vi "Z900_navX_Internal_Open.vi"(8 "error in":errorcluster, 11 "navX Device":T1={"Interface"={"Protocol"=enum."SERIAL", "Update Rate (4Hz-60Hz)"=4, "navX Open TypeDef"=variant}, "Notify Packet"=refnum, "Loop VI Refnum"=refnum, "Ready to Close Occurrence Refnum"=refnum} {"Interface"."Update Rate (4Hz-60Hz)" min=4 max=60 step=1}) -> (0 "error out":errorcluster, 2 "Interface TypeDefs":T3 {"I2CDevRef"."Device Address" format="%.0x"}, 3 "navX Device":T1={"Interface"={"Protocol"=enum."SERIAL", "Update Rate (4Hz-60Hz)"=4, "navX Open TypeDef"=variant}, "Notify Packet"=refnum, "Loop VI Refnum"=refnum, "Ready to Close Occurrence Refnum"=refnum} {"Interface"."Update Rate (4Hz-60Hz)" min=4 max=60 step=1})   [LabVIEW 2016, in "navX Library v2.lvlib"]
doc: "This navX VI handles opening the Serial/I2C/SPI reference for the navX.\nTHIS VI SHOULD NOT BE CALLED BY THE USER!"
uses:
  navX Library v2.lvlib
  TypeDefs/Z900_navX_DeviceTypeDef.ctl
  TypeDefs/Z900_navX_ProtocolTypeDef.ctl
  TypeDefs/Z900_navX_NotifyPacketTypeDef.ctl
  TypeDefs/Z900_navX_ActionTypeDef.ctl
  TypeDefs/Z900_navX_InterfaceTypeDef.ctl
  <vilib>/Rock Robotics/WPI/SerialPort/WPI_SerialPortRef.ctl
  <vilib>/Rock Robotics/WPI/I2C/WPI_I2CDevRef.ctl
  <vilib>/Rock Robotics/SystemInterfaces/i2clib/i2c_bus.ctl
  <vilib>/Rock Robotics/WPI/SPI/WPI_SPIDevRef.ctl
  <vilib>/Rock Robotics/SystemInterfaces/spilib/spi_bus.ctl
  TypeDefs/navX Open TypeDefs/Z900_navX_OpenTypeDef_Serial.ctl
  NI WPI/WPI_SerialPort_USB.ctl
  TypeDefs/Z900_navX_SerialStreamTypeDef.ctl
  TypeDefs/navX Open TypeDefs/Z900_navX_OpenTypeDef_I2C.ctl
  TypeDefs/navX Open TypeDefs/Z900_navX_OpenTypeDef_SPI.ctl
  NI WPI/NI WPI Serial USB.lvlib
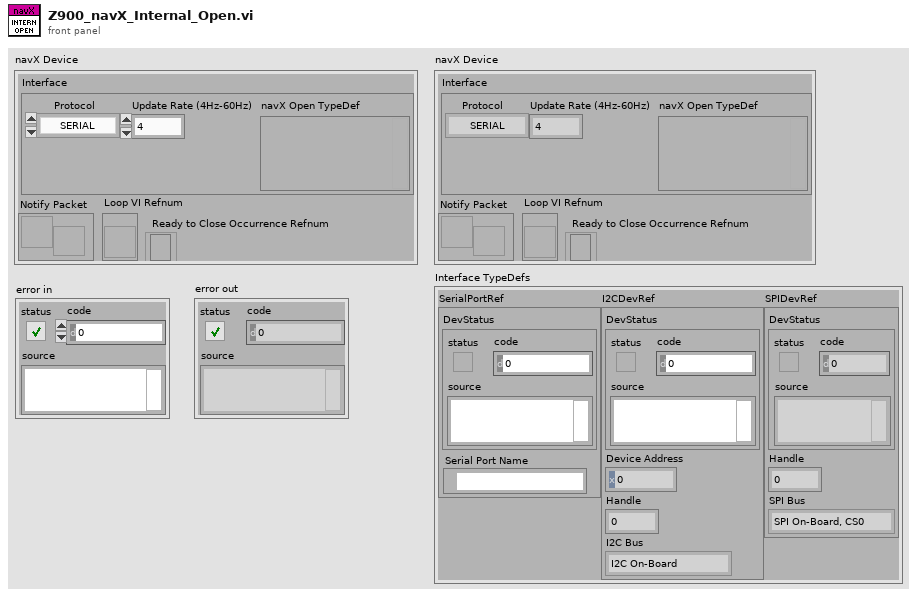
[diagram p1: front panel]
types:
  T1 = typedef "navX Library v2.lvlib/Z900_navX_DeviceTypeDef.ctl" = cluster{"Interface":cluster{"Protocol":T2, "Update Rate (4Hz-60Hz)":u8, "navX Open TypeDef":variant}, "Notify Packet":refnum<notifier>, "Loop VI Refnum":refnum<vi>, "Ready to Close Occurrence Refnum":refnum<k4>}
  T2 = typedef "navX Library v2.lvlib/Z900_navX_ProtocolTypeDef.ctl" = enum16{"SERIAL", "I2C", "SPI"}
  T3 = typedef "navX Library v2.lvlib/Z900_navX_InterfaceTypeDef.ctl" = cluster{"SerialPortRef":T4, "I2CDevRef":T5, "SPIDevRef":T7}
  T4 = typedef "WPI_SerialPortRef.ctl" = cluster{"DevStatus":errorcluster, "Serial Port Name":refnum<visa-resource-name>}
  T5 = typedef "WPI_I2CDevRef.ctl" = cluster{"DevStatus":errorcluster, "Device Address":u8, "Handle":i32, "I2C Bus":T6}
  T6 = typedef "i2c_bus.ctl" = enum16{"I2C On-Board", "I2C MXP", "Invalid"}
  T7 = typedef "WPI_SPIDevRef.ctl" = cluster{"DevStatus":errorcluster, "Handle":i32, "SPI Bus":T8}
  T8 = typedef "spi_bus.ctl" = enum16{"SPI On-Board, CS0", "SPI On-Board, CS1", "SPI On-Board, CS2", "SPI On-Board, CS3", "SPI MXP", "Invalid"}
  T9 = typedef "navX Library v2.lvlib/Z900_navX_OpenTypeDef_Serial.ctl" = cluster{"Serial Port":T10, "Stream Type":T11}
  T10 = typedef "NI WPI Serial USB.lvlib/WPI_SerialPort_USB.ctl" = enum16{"Onboard RS-232", "MXP TTL", "USB"}
  T11 = typedef "navX Library v2.lvlib/Z900_navX_SerialStreamTypeDef.ctl" = enum16{"YRPH", "Quaterinons", "Gyro/Raw", "AHRS", "AHRSAndPositioning"}
  T12 = typedef "navX Library v2.lvlib/Z900_navX_OpenTypeDef_I2C.ctl" = cluster{"I2C Bus":T6}
  T13 = typedef "navX Library v2.lvlib/Z900_navX_OpenTypeDef_SPI.ctl" = cluster{"SPI Bus":T8, "Clock Rate (Hz)":dbl}
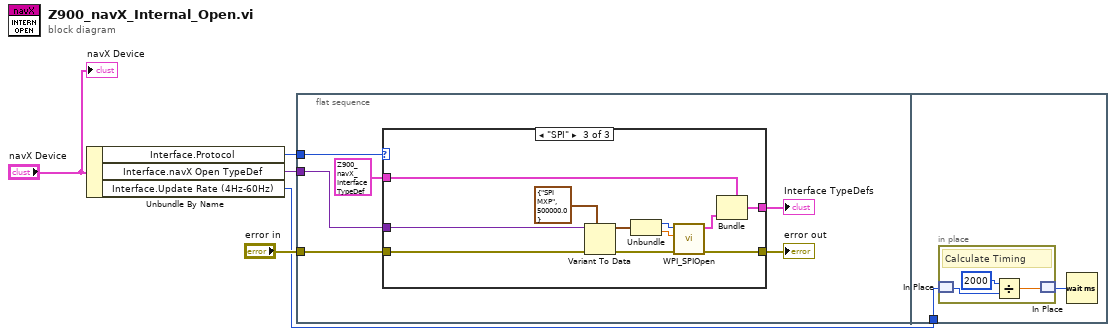
[diagram p0: block diagram]
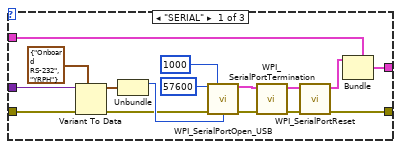
[diagram p2: hidden frame]
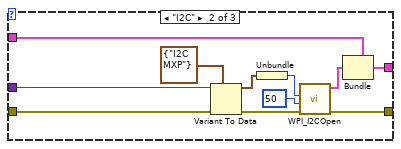
[diagram p3: hidden frame]
diagram:
  n1 = Unbundle By Name("navX Device") -> ("Interface.Protocol"=w5:T2, "Interface.navX Open TypeDef"=w4:variant, "Interface.Update Rate (4Hz-60Hz)"=w1:u8)
  n2 = flat-sequence {
    tunnel: w5 -> [w11]
    tunnel: w4 -> [w10]
    tunnel: "error in" -> [w8]
    tunnel: w1 -> [w50]
    frame #0 {
      n3 = case shown="\"SPI\"" w11 {
        tunnel: w10 -> [w27 w37 w48]
        tunnel: [w19 w33 w45] -> w9
        tunnel: w8 -> [w18 w31 w44]
        tunnel: T3 {"SerialPortRef"={"DevStatus"={"status"=FALSE, "code"=0, "source"=""}, "Serial Port Name"=""}, "I2CDevRef"={"DevStatus"={"status"=FALSE, "code"=0, "source"=""}, "Device Address"=0, "Handle"=0, "I2C Bus"=enum."I2C On-Board"}, "SPIDevRef"={"DevStatus"={"status"=FALSE, "code"=0, "source"=""}, "Handle"=0, "SPI Bus"=enum."SPI On-Board, CS0"}} ("Interface TypeDefs") -> [w15 w30 w42]
        tunnel: [w16 w29 w40] -> w6
        frame "SERIAL" {
          n4 = Variant To Data(error in=w18, type=T9 {"Serial Port"=enum."Onboard RS-232", "Stream Type"=enum."YRPH"} ("navX Serial Open"), Variant=w27) -> (data=w25:T9, error out=w17:errorcluster)
          n5 = Unbundle(w25) -> ("Serial Port"=w24:T10)  [unwired: 1 out]
          n6 = call "WPI_SerialPortOpen_USB.vi"("Baud Rate"=u32 57600, "Timeout Value (ms)"=u32 1000, "error in (no error)"=w17, "Serial Port"=w24) -> ("SerialPortRef"=w21:T4, "error out"=w20:errorcluster)  [unwired: 10 in]
          n7 = call <vilib>:"WPI_SerialPortTermination.vi"("error in (no error)"=w20, "SerialPortRef"=w21) -> ("error out"=w12:errorcluster, "SerialPortRef"=w13:T4)  [unwired: 8 in]
          n8 = call <vilib>:"WPI_SerialPortReset.vi"("error in (no error)"=w12, "SerialPortRef"=w13) -> ("error out"=w19:errorcluster, "SerialPortRef"=w14:T4)  [unwired: 8 in]
          n9 = Bundle(cluster=w15, "SerialPortRef"=w14) -> (w16:T3)  [unwired: 2 in]
        }
        frame "I2C" {
          n10 = Variant To Data(error in=w31, type=T12 {"I2C Bus"=enum."I2C MXP"} ("navX I2C Open"), Variant=w37) -> (data=w38:T12, error out=w32:errorcluster)
          n11 = Unbundle(w38) -> ("I2C Bus"=w35:T6)
          n12 = call <vilib>:"WPI_I2COpen.vi"("error in"=w32, "Device Address"=u8 50, "I2C Bus"=w35) -> ("error out"=w33:errorcluster, "I2CDevRef"=w28:T5)  [unwired: 7 in]
          n13 = Bundle(cluster=w30, "I2CDevRef"=w28) -> (w29:T3)  [unwired: 2 in]
        }
        frame "SPI" {
          n14 = Variant To Data(error in=w44, type=T13 {"SPI Bus"=enum."SPI MXP", "Clock Rate (Hz)"=500000.0} ("navX SPI Open"), Variant=w48) -> (data=w49:T13, error out=w43:errorcluster)
          n15 = Unbundle(w49) -> ("SPI Bus"=w46:T8, "Clock Rate (Hz)"=w39:dbl)
          n16 = call <vilib>:"WPI_SPIOpen.vi"("error in"=w43, "Clock Rate (Hz)"=w39, "SPI Bus"=w46) -> ("error out"=w45:errorcluster, "SPIDevRef"=w41:T7)  [unwired: 7 in]
          n17 = Bundle(cluster=w42, "SPIDevRef"=w41) -> (w40:T3)  [unwired: 2 in]
        }
      }
      "Interface TypeDefs" <- w6
      "error out" <- w9
    }
    frame #1 {
      n18 = in-place {
        # "Calculate Timing"
        n19 = in-place-match #1(w50) -> (w53:u8)
        n20 = Divide(x=2000, y=w53) -> (x/y=w52:dbl)
        n21 = in-place-match #1(w52) -> (w51:u8)
      }
      n22 = Wait (ms)(milliseconds to wait=w51) -> ()  [unwired: 1 out]
    }
  }
  "navX Device" <- "navX Device"
